vi "Graph.vi"(6 "Array":dbl[](array[numeric]), 9 "Частота (1000 Hz)":dbl, 10 "Количество точек":dbl, 11 "Амплитуда":dbl) -> (2 "XY Graph 3":cluster{"Y":dbl[], "Y":dbl[]}[](graph))   [LabVIEW 2012]
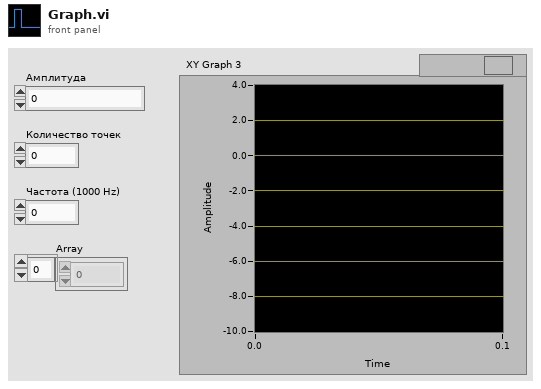
[diagram p1: front panel]
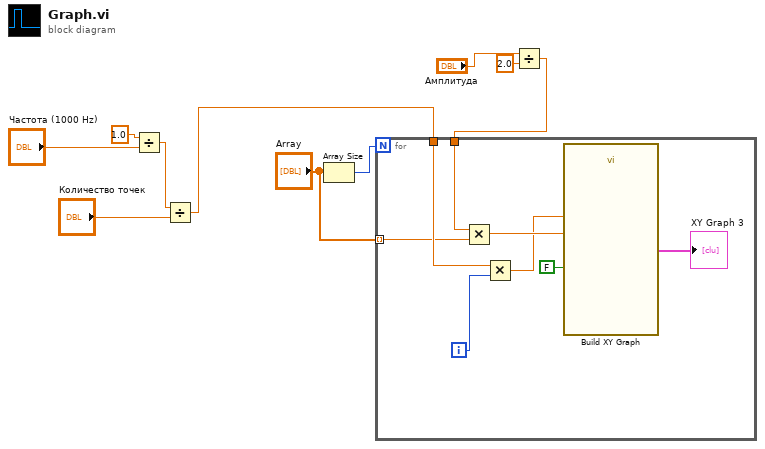
[diagram p0: block diagram]
diagram:
  n1 = Divide(x=1.0, y="Частота (1000 Hz)") -> (x/y=w7:dbl)
  n2 = Divide(x=w7, y="Количество точек") -> (x/y=w8:dbl)
  n3 = Array Size(array="Array") -> (size(s)=w5:i32)
  n4 = Divide(x="Амплитуда", y=2.0) -> (x/y=w1:dbl)
  n5 = for {
    N: w5 -> [_]
    tunnel: "Array" -> [w13] mode=indexing
    tunnel: w1 -> [w12]
    tunnel: w8 -> [w15]
    i -> [w14]
    n6 = Multiply(x=w12, y=w13) -> (x*y=w17:dbl)
    n7 = Multiply(x=w15, y=w14) -> (x*y=w16:dbl)
    n8 = call "Build XY Graph"("Reset"=FALSE, "Y Input"=w17, "X Input"=w16) -> ("XY Graph"=→"XY Graph 3":cluster{"Y":dbl[], "Y":dbl[]}[])  [unwired: 2 in, 6 out]
  }
